vi "基础队列INI.vi"(8 "error in (no error)":errorcluster caption="错误输入（无错误）", 11 "MainPage 输入":refnum<class "MainPage.lvclass">) -> (0 "error out":errorcluster caption="错误输出", 3 "MainPage 输出":refnum<class "MainPage.lvclass">)   [LabVIEW 2019, in "MainPage.lvlib" / "MainPage.lvclass"]
uses:
  MainPage.lvclass
  MainPage.lvclass/MainPage.ctl
panel:
  # "主要用于通讯模块动作通知队列\n和报文发送队列（排序及存储）\n的创建队列，方便后续程序中调用使用"
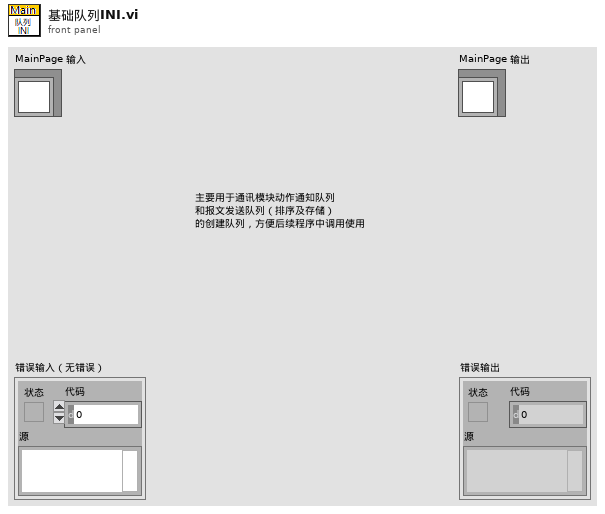
[diagram p1: front panel]
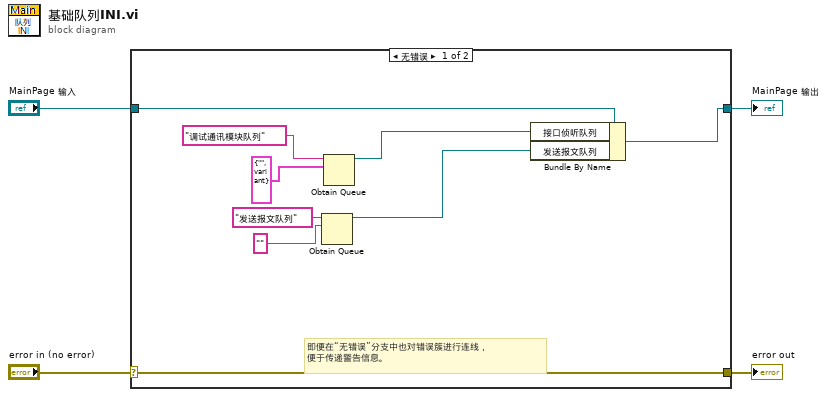
[diagram p0: block diagram]
diagram:
  n1 = case shown="无错误" "error in (no error)" {
    selector: "error in (no error)" -> [w13 w15]
    tunnel: [w13 w15] -> w3
    tunnel: [w9 w14] -> w1
    tunnel: "MainPage 输入" -> [w10 w14]
    frame No Error {
      # "即便在“无错误”分支中也对错误簇进行连线，\n便于传递警告信息。"
      n2 = Obtain Queue(name (unnamed)="发送报文队列" ("名称（未命名）"), element data type="") -> (queue out=w7:refnum<queue>)  [unwired: 3 in, 2 out]
      n3 = Obtain Queue(name (unnamed)="调试通讯模块队列" ("名称（未命名）"), element data type=cluster{string, variant} {"", variant}) -> (queue out=w8:refnum<queue>)  [unwired: 3 in, 2 out]
      n4 = Bundle By Name(cluster=w10, "接口侦听队列"=w8, "发送报文队列"=w7) -> (w9:refnum<class "MainPage.lvclass">)
    }
    frame Error {
    }
  }
  "error out" <- w3
  "MainPage 输出" <- w1
